vi "ZCAN_IsDeviceOnline.vi"(8 "error in (no error)":errorcluster caption="错误输入（无错误）", 10 "device_handle":u64) -> (0 "error out":errorcluster caption="错误输出", 2 "Online?":bool)   [LabVIEW 2018, in "zlgcan.lvlib"]
doc: "该函数用于关闭设备，关闭设备和打开设备一一对应。\n\n调用该函数，会关闭整个CAN设备（对于设备句柄），不分通道。"
uses:
  zlgcan.lvlib
  bin/ControlCANFD.dll
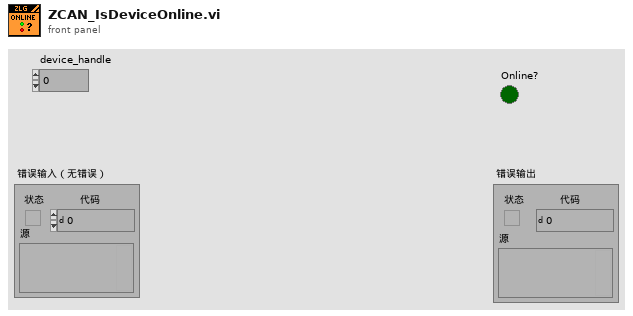
[diagram p1: front panel]
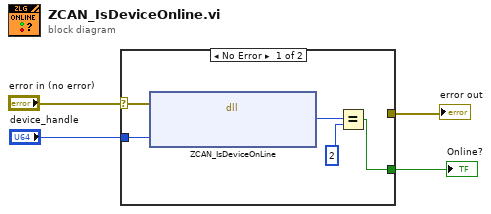
[diagram p0: block diagram]
diagram:
  n1 = case shown="No Error" "error in (no error)" {
    selector: "error in (no error)" -> [w5 w10]
    tunnel: [_ w10] -> w3
    tunnel: "device_handle" -> [w9 _]
    tunnel: [w6 _] -> w1
    frame No Error {
      n2 = dll-call lib="C:/Users/ttc52/Desktop/DHC FD LV2018/LABIVIEW CANFD Tool_V1.2.4_20220724/bin/ControlCANFD.dll" fn="ZCAN_IsDeviceOnLine" ("ZCAN_StartCAN")(error in=w5, "device_handle"=w9) -> ("return"=w7:u32)  [unwired: 3 in, 2 out]
      n3 = Equal?(x=w7, y=u32 2) -> (x = y?=w6:bool)
    }
    frame Error {
    }
  }
  "error out" <- w3
  "Online?" <- w1
